vi "Pfeiffer Vacuum HLT5xx Operating Turbopump.vi"(8 "error in (no error)":errorcluster, 9 "Operating adjustment - Cluster":T1={"Parameter"=0, "Parameter\nread only<->describe"=FALSE, "Motor Turbopump\noff<->on"=TRUE, "End of measuring\nrange of gauge"=0} {"End of measuring\nrange of gauge" items=[" 0,1 mbar", " 1 mbar", " 10 mbar", " 100 mbar", " 1000 mbar", " 2000 mbar", " 5000 mbar", " 10000 mbar", " 50000 mbar"]; "Parameter" items=[" End of measuring range of gauge", " Motor Turbopump", " Actual rotation speed TMP [Hz] (read only)", " Motor current TMP [A] (read only)", " Software version electronic drive unit  (read only)", " Operating hours TMP [h] (read only)", " Unit type electronic drive unit (read only)"]}, 10 "Adress of unit":u16=1 min=1 max=999 step=1, 11 "COM Port Name in":refnum<visa-resource-name>="COM1") -> (0 "error out":errorcluster, 3 "response (data)":string)   [LabVIEW 2016]
doc: "This VI is an example of how to use the Pfeiffer Vacuum subVIs programmatically. This VI first initializes the instrument, takes measurements, then closes the instrument."
uses:
  Public/LeakDetector/PV HLT5xx Operating Turbopump - Cluster.ctl
  Pfeiffer Vacuum.lvlib
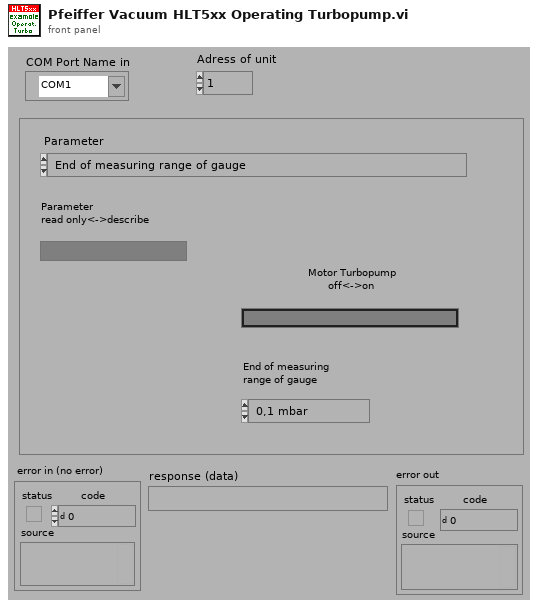
[diagram p1: front panel]
types:
  T1 = typedef "Pfeiffer Vacuum.lvlib/PV HLT5xx Operating Turbopump - Cluster.ctl" = cluster{"Parameter":u16, "Parameter\nread only<->describe":bool, "Motor Turbopump\noff<->on":bool, "End of measuring\nrange of gauge":u16}
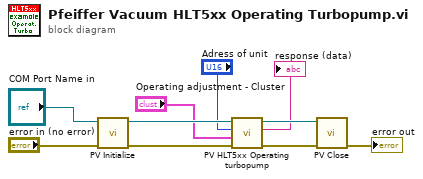
[diagram p0: block diagram]
diagram:
  n1 = call "PV Initialize.vi"("error in (no error)"="error in (no error)", "VISA session in"="COM Port Name in") -> ("error out"=w10:errorcluster, "VISA session out"=w8:refnum<visa-resource-name>)  [unwired: 8 in]
  n2 = call "PV HLT5xx Operating turbopump.vi"("error in (no error)"=w10, "Operating adjustment - Cluster"="Operating adjustment - Cluster", "Adress of unit"="Adress of unit", "VISA session"=w8) -> ("error out"=w9:errorcluster, "response (data)"=→"response (data)":string, "dup VISA session"=w7:refnum<visa-resource-name>)  [unwired: 5 in]
  n3 = call "PV Close.vi"("VISA session"=w7, "error in (no error)"=w9) -> ("error out"=→"error out":errorcluster)  [unwired: 13 in]
